vi "Read Key (String).vi"(6 "read raw string? (F)":bool, 7 "section":string, 8 "error in (no error)":errorcluster, 9 "default value":string, 10 "key":string, 11 "refnum":T1) -> (0 "error out":errorcluster, 1 "value":string, 2 "found?":bool, 3 "refnum out":T1)   [LabVIEW 2017]
doc: "Reads a value associated with a key in a specified section from the configuration data identified by <B>refnum</B>. If the key does not exist, the VI returns the default value. This VI supports multibyte characters in strings. Wire data to the <B>default value</B> input to determine the polymorphic instance to use or manually select the instance."
uses:
  DSFConfig.lvlib
  DSF Config Data RefNum.ctl
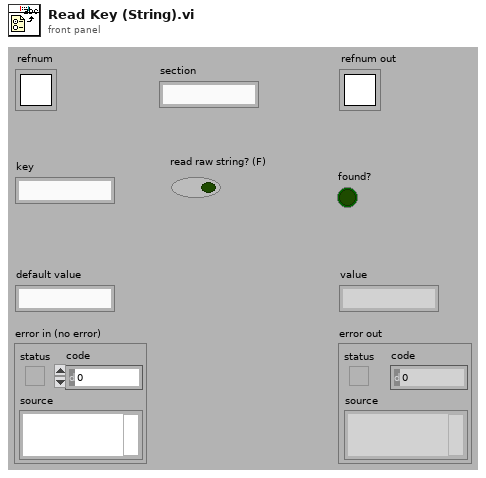
[diagram p1: front panel]
types:
  T1 = typedef "DSFConfig.lvlib/DSF Config Data RefNum.ctl" = refnum<k1>
  T2 = typedef "DSFConfig.lvlib/Config Queue.ctl" = refnum<queue>
  T3 = typedef "DSFConfig.lvlib/Config Data.ctl" = cluster{"dsf configuration":T4, "path":path, "dirty":bool}
  T4 = typedef "DSFConfig.lvlib/DSF Config.ctl" = cluster{"dsf":T5, "configuration":T5, "plugins":T6[], "groups":T9[], "transfers":T11[], "channels":T13[], "settings":T15[]}
  T5 = typedef "DSFConfig.lvlib/Version Info.ctl" = cluster{"major":u32, "minor":u32, "fix":u32, "build":string}
  T6 = typedef "DSFConfig.lvlib/DSF Plugin.ctl" = cluster{"id":string, "values":T7}
  T7 = typedef "DSFConfig.lvlib/DSF Plugin Info.ctl" = cluster{"type":string, "timing":T8, "group ids":string[], "settings id":string}
  T8 = typedef "DSFConfig.lvlib/DSF Timing Info.ctl" = cluster{"decimation":i32, "offset":i32}
  T9 = typedef "DSFConfig.lvlib/DSF Group.ctl" = cluster{"id":string, "values":T10}
  T10 = typedef "DSFConfig.lvlib/DSF Group Info.ctl" = cluster{"direction":i32, "timing":T8, "transfer ids":string[], "settings id":string}
  T11 = typedef "DSFConfig.lvlib/DSF Transfer.ctl" = cluster{"id":string, "values":T12}
  T12 = typedef "DSFConfig.lvlib/DSF Transfer Info.ctl" = cluster{"byte order":i32, "channel ids":string[], "settings id":string}
  T13 = typedef "DSFConfig.lvlib/DSF Channel.ctl" = cluster{"id":string, "values":T14}
  T14 = typedef "DSFConfig.lvlib/DSF Channel Info.ctl" = cluster{"count":i32, "offset":i32, "data type":i32, "resource path":string, "settings id":string}
  T15 = typedef "DSFConfig.lvlib/DSF Settings.ctl" = cluster{"id":string, "values":T16}
  T16 = typedef "DSFConfig.lvlib/DSF Settings Info.ctl" = cluster{"key":string, "value":string}[]
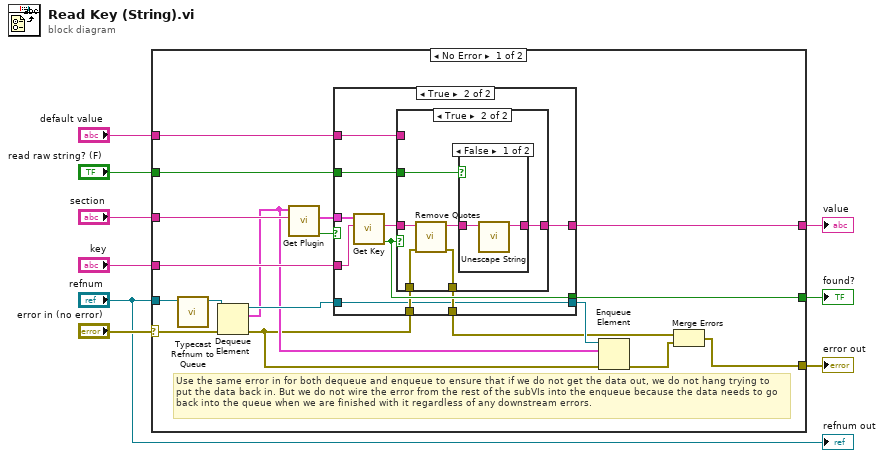
[diagram p0: block diagram]
diagram:
  n1 = case shown="No Error" "error in (no error)" {
    selector: "error in (no error)" -> [w21 w53]
    tunnel: [w11 w53] -> w8
    tunnel: "refnum" -> [w23 _]
    tunnel: "section" -> [w20 _]
    tunnel: "key" -> [w17 _]
    tunnel: "default value" -> [w27 w52]
    tunnel: [w25 _] -> w5
    tunnel: [w26 w52] -> w3
    tunnel: "read raw string? (F)" -> [w24 _]
    frame No Error {
      # "Use the same error in for both dequeue and enqueue to ensure that if we do not get the data out, we do not hang trying to put the data back in. But we do not wire the error from the rest of the subVIs into the enqueue because the data needs to go back into the queue when we are finished with it regardless of any downstream errors."
      n2 = call "Typecast Refnum to Queue.vi"("refnum in"=w23) -> ("queue out"=w22:T2)  [unwired: 10 in]
      n3 = Dequeue Element(queue=w22, error in (no error)=w21) -> (queue out=w16:T2, element=w14:T3, error out=w10:errorcluster)  [unwired: 1 in, 1 out]
      n4 = call "Get Plugin.vi"("id"=w20, "element"=w14) -> ("exists?"=w19:bool, "info"=w18:T7)  [unwired: 6 in, 2 out]
      n5 = case shown="True" w19 {
        tunnel: w27 -> [w30 w40]
        tunnel: [w30 w39] -> w26
        tunnel: [_ w35] -> w25
        tunnel: w24 -> [_ w38]
        tunnel: w18 -> [_ w37]
        tunnel: w17 -> [_ w36]
        tunnel: w10 -> [w29 w33]
        tunnel: [w29 w32] -> w13
        tunnel: w16 -> [w28 w31]
        tunnel: [w28 w31] -> w15
        frame False {
          # "use default value"
        }
        frame True {
          n6 = call "Get Key.vi"("key"=w36, "section data"=w37) -> ("key exists?"=w35:bool, "value"=w34:string)  [unwired: 5 in, 3 out]
          n7 = case shown="True" w35 {
            tunnel: w40 -> [w42 _]
            tunnel: [w42 w48] -> w39
            tunnel: w38 -> [_ w47]
            tunnel: w34 -> [_ w45]
            tunnel: w33 -> [w41 w44]
            tunnel: [w41 w43] -> w32
            frame False {
              # "use default value"
            }
            frame True {
              n8 = call "Remove Quotes.vi"("error in (no error)"=w44, "string"=w45) -> ("error out"=w43:errorcluster, "without quotes"=w46:string)  [unwired: 7 in, 1 out]
              n9 = case shown="False" w47 {
                tunnel: [w50 w51] -> w48
                tunnel: w46 -> [w49 w51]
                frame False {
                  n10 = call "Unescape String.vi"("string"=w49) -> ("parsed string"=w50:string)  [unwired: 10 in]
                }
                frame True {
                }
              }
            }
          }
        }
      }
      n11 = Enqueue Element(queue=w15, element=w14, error in (no error)=w10) -> (error out=w12:errorcluster)  [unwired: 1 in, 2 out]
      n12 = Merge Errors(w13, w12) -> (w11:errorcluster)
    }
    frame Error {
    }
  }
  "error out" <- w8
  "found?" <- w5
  "value" <- w3
  "refnum out" <- "refnum"
